vi "DisconnectBkPrecision.vi"(1 "error out":errorcluster, 2 "VISA resource name out":refnum<visa-resource-name>) -> ()   [LabVIEW 2010]
uses:
  <instrlib>/BK Precision 85XX Series/BK Precision 85XX Series.lvlib
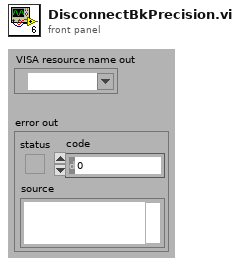
[diagram p1: front panel]
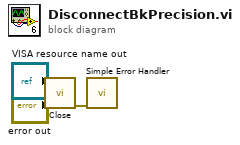
[diagram p0: block diagram]
diagram:
  n1 = call <instrlib>:"Close.vi"("error in (no error)"="error out", "VISA resource name"="VISA resource name out") -> ("error out"=w1:errorcluster)  [unwired: 9 in]
  n2 = call <vilib>:"Simple Error Handler.vi"("error in (no error)"=w1) -> ()  [unwired: 4 in, 5 out]
